vi "Coerce-table-value.vi"(0 "Y":i32, 1 "X":i32, 2 "Z":i32, 3 "P":i32) -> (4 "In range ?":bool, 5 "coerced Y":i32, 6 "coerced X":i32, 7 "coerced Z":i32, 8 "coerced P":i32)   [LabVIEW 2019]
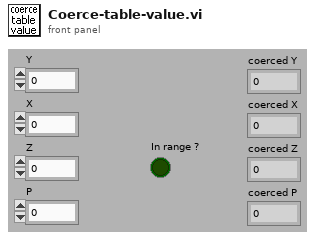
[diagram p1: front panel]
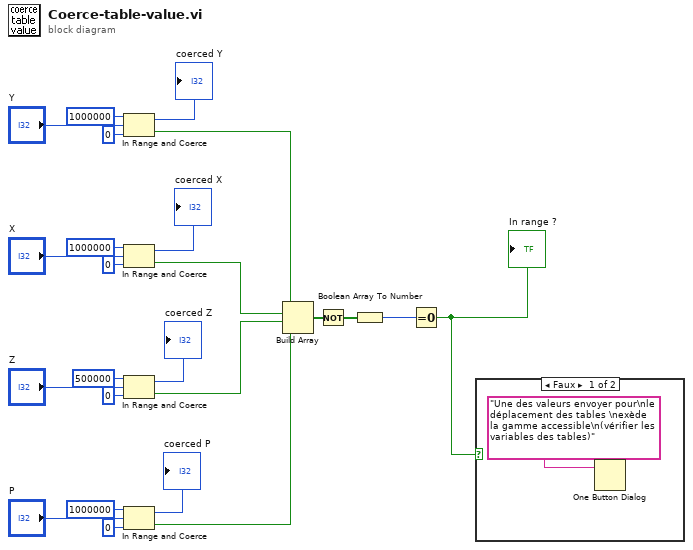
[diagram p0: block diagram]
diagram:
  n1 = In Range and Coerce(upper limit=1000000, x="Y", lower limit=0) -> (coerced(x)=→"coerced Y":i32, In Range?=w19:bool)
  n2 = In Range and Coerce(upper limit=1000000, x="X", lower limit=0) -> (coerced(x)=→"coerced X":i32, In Range?=w18:bool)
  n3 = In Range and Coerce(upper limit=500000, x="Z", lower limit=0) -> (coerced(x)=→"coerced Z":i32, In Range?=w17:bool)
  n4 = In Range and Coerce(upper limit=1000000, x="P", lower limit=0) -> (coerced(x)=→"coerced P":i32, In Range?=w16:bool)
  n5 = Build Array(w19, w18, w17, w16) -> (w20:bool[])
  n6 = Not(x=w20) -> (.not. x?=w3:bool[])
  n7 = Boolean Array To Number(Boolean array=w3) -> (number=w15:u32)
  n8 = Equal To 0?(x=w15) -> (x = 0?=w4:bool)
  "In range ?" <- w4
  n9 = case shown="Faux" w4 {
    frame False {
      n10 = One Button Dialog(message="Une des valeurs envoyer pour\nle déplacement des tables \nexède la gamme accessible\n(vérifier les variables des tables)") -> ()  [unwired: 1 in, 1 out]
    }
    frame True {
    }
  }
